vi "DriveStraightDistance.vi"(10 "desiredDistance":dbl, 11 "DriveBase.lvclass":refnum<class "DriveBase.lvclass">) -> (3 "DriveBase.lvclass 2":refnum<class "DriveBase.lvclass">)   [LabVIEW 2016, in "DriveBase.lvclass"]
uses:
  DriveBase.lvclass
panel:
  in  "desiredDistance 2":dbl
  out "DriveBase.lvclass 4":refnum<class "DriveBase.lvclass">
  in  "DriveBase.lvclass 3":refnum<class "DriveBase.lvclass">
  # "Disabled"
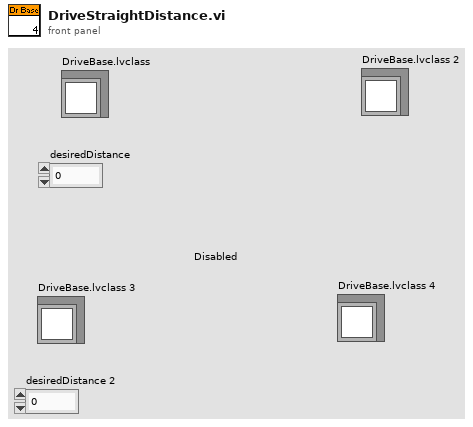
[diagram p1: front panel]
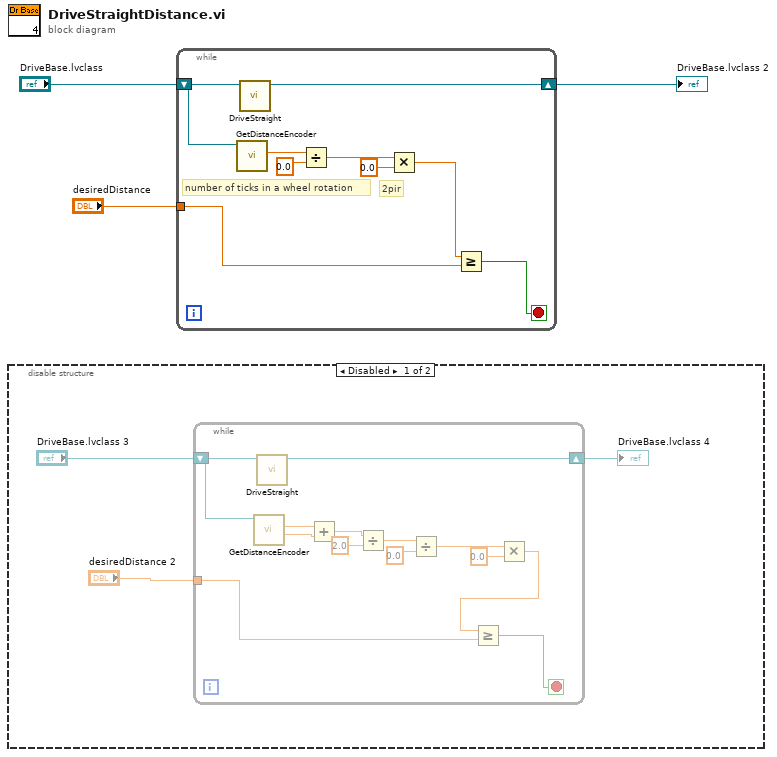
[diagram p0: block diagram]
diagram:
  n1 = disable-structure shown="Disabled" {
    frame Disabled {
      n2 = while {
        shift-right: [w19] -> w5
        shift-left: "DriveBase.lvclass 3" -> [w16]
        tunnel: "desiredDistance 2" -> [w17]
        stop <- w18 stop-if-true
        n3 = call "GetDistanceEncoder.vi"("DriveBase.lvclass"=w16) -> ("leftDistanceEncoderOutput"=w11:dbl, "rightDistanceEncoderOutput"=w12:dbl)  [unwired: 8 in, 1 out]
        n4 = call "DriveStraight.vi"("DriveBase.lvclass"=w16) -> ("DriveBase.lvclass 2"=w19:refnum<class "DriveBase.lvclass">)  [unwired: 10 in]
        n5 = Add(x=w12, y=w11) -> (x+y=w10:dbl)
        n6 = Divide(x=w10, y=2.0) -> (x/y=w8:dbl)
        n7 = Divide(x=w8, y=0.0) -> (x/y=w14:dbl)
        n8 = Multiply(x=w14, y=0.0) -> (x*y=w7:dbl)
        n9 = Greater Or Equal?(x=w7, y=w17) -> (x >= y?=w18:bool)
      }
      "DriveBase.lvclass 4" <- w5
    }
    frame Enabled {
    }
  }
  n10 = while {
    shift-right: [w28] -> w2
    shift-left: "DriveBase.lvclass" -> [w25]
    tunnel: "desiredDistance" -> [w26]
    stop <- w27 stop-if-true
    # "2pir"
    # "number of ticks in a wheel rotation"
    n11 = call "GetDistanceEncoder.vi"("DriveBase.lvclass"=w25) -> ("rightDistanceEncoderOutput"=w24:dbl)  [unwired: 8 in, 2 out]
    n12 = call "DriveStraight.vi"("DriveBase.lvclass"=w25) -> ("DriveBase.lvclass 2"=w28:refnum<class "DriveBase.lvclass">)  [unwired: 10 in]
    n13 = Divide(x=w24, y=0.0) -> (x/y=w22:dbl)
    n14 = Multiply(x=w22, y=0.0) -> (x*y=w20:dbl)
    n15 = Greater Or Equal?(x=w20, y=w26) -> (x >= y?=w27:bool)
  }
  "DriveBase.lvclass 2" <- w2
